vi "32Bit_SignExtend Single.vi"(8 "Data In":u32, 9 "# data bits":i8) -> (0 "I32 data":i32 caption="I32 data (sign extended)")   [LabVIEW 2010, in "lib1299.lvlib"]
uses:
  lib1299.lvlib
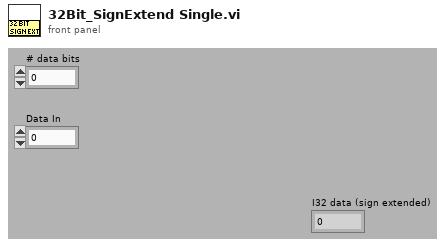
[diagram p1: front panel]
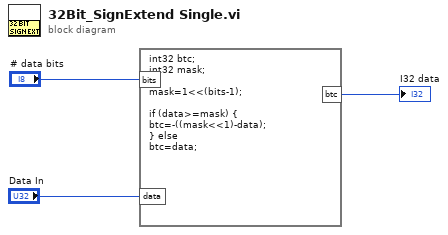
[diagram p0: block diagram]
diagram:
  n1 = formula code="int32 btc;\nint32 mask;\n\nmask=1<<(bits-1);\n\nif (data>=mask) {\nbtc=-((mask<<1)-data);\n} else\nbtc=data;"("bits"="# data bits", "data"="Data In") -> ("btc"=→"I32 data":i32)
